vi "rywindow_test.vi"() -> ()   [LabVIEW 2017]
uses:
  rywindow.lvclass
panel:
  in  "Multicolumn Listbox":i32(listbox)
  out "error out":errorcluster
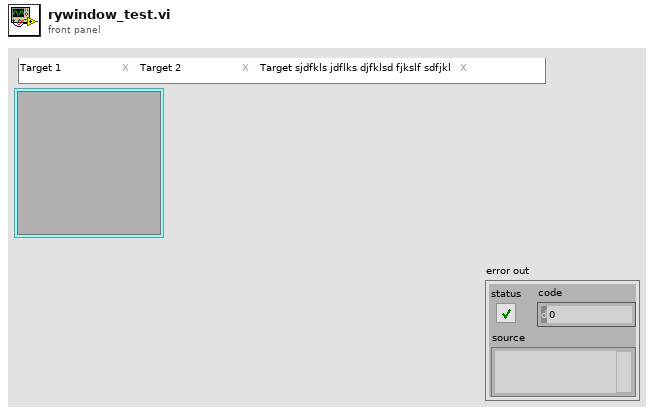
[diagram p1: front panel]
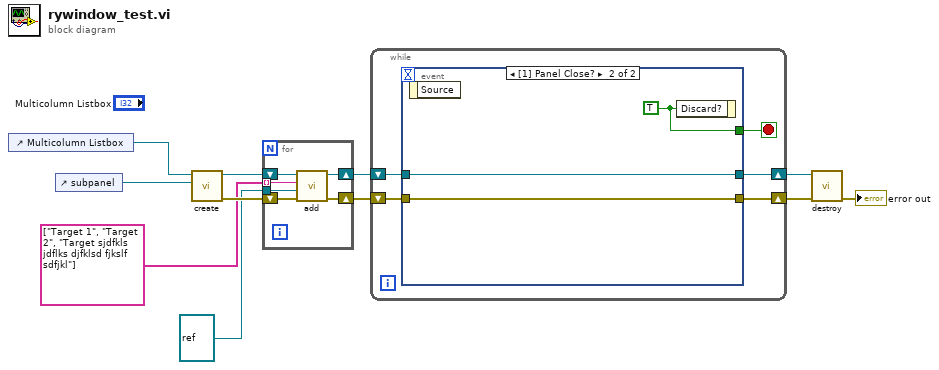
[diagram p0: block diagram]
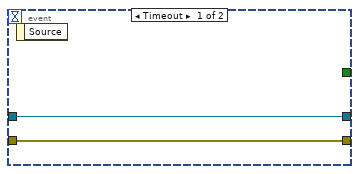
[diagram p2: hidden frame]
diagram:
  n1 = control-ref of="Multicolumn Listbox"() -> (w1:refnum<vi>)
  n2 = control-ref of="subpanel"() -> (w11:refnum<vi>)
  n3 = call "create.vi"("subpanel"=w11, "mclb"=w1) -> ("error out"=w10:errorcluster, "window"=w9:refnum<class "rywindow.lvclass">)  [unwired: 8 in]
  n4 = for {
    tunnel: string[] ["Target 1", "Target 2", "Target sjdfkls jdflks djfklsd fjkslf sdfjkl"] -> [w15] mode=indexing
    tunnel: refnum<vi> refnum ("vi refnum") -> [w14]
    shift-right: [w13] -> w6
    shift-left: w10 -> [w17]
    shift-right: [w12] -> w5
    shift-left: w9 -> [w16]
    n5 = call "add.vi"("error in (no error)"=w17, "vi refnum"=w14, "name"=w15, "window in"=w16) -> ("error out"=w13:errorcluster, "window out"=w12:refnum<class "rywindow.lvclass">)  [unwired: 6 in]
  }
  n6 = while {
    shift-right: [w20] -> w3
    shift-left: w5 -> [w21]
    shift-right: [w19] -> w4
    shift-left: w6 -> [w18]
    stop <- w22 stop-if-true
    n7 = event shown="[1] Panel Close?" {
      selector: _ -> [_ _]
      dyn-events: _ -> [_ _]
      timeout: _ -> [_ _]
      tunnel: [_ w27] -> w22
      tunnel: w21 -> [w23 w26]
      tunnel: [w23 w26] -> w20
      tunnel: [w24 w25] -> w19
      tunnel: w18 -> [w24 w25]
      event Timeout {
        n8 = event-data() -> ()  [unwired: 1 in, 1 out]
      }
      event Panel Close? {
        w27 = TRUE ("Discard?")
        n9 = event-data() -> ()  [unwired: 1 in, 1 out]
        n10 = event-data("Discard?"=w27) -> ()  [unwired: 1 in, 1 out]
      }
    }
  }
  n11 = call "destroy.vi"("error in (no error)"=w4, "window"=w3) -> ("error out"=→"error out":errorcluster)  [unwired: 9 in]
